vi "Class Loading Progress.vi"(8 "error in (no error)":errorcluster, 10 "Progress (%)":T1 scale=0.0..100.0, 11 "Test Caller Actor in":refnum<class "Test Caller Actor.lvclass">) -> (0 "error out":errorcluster, 3 "Test Caller Actor out":refnum<class "Test Caller Actor.lvclass">)   [LabVIEW 2023, in "Test Caller Actor.lvlib" / "Test Caller Actor.lvclass"]
uses:
  Test Caller Actor.lvclass
  Test Caller Actor.lvclass/Test Caller Actor.ctl
  Class Loader/Class Loader/Loading Progress.ctl
  Class Loader/Class Loader/Class Loader.lvclass
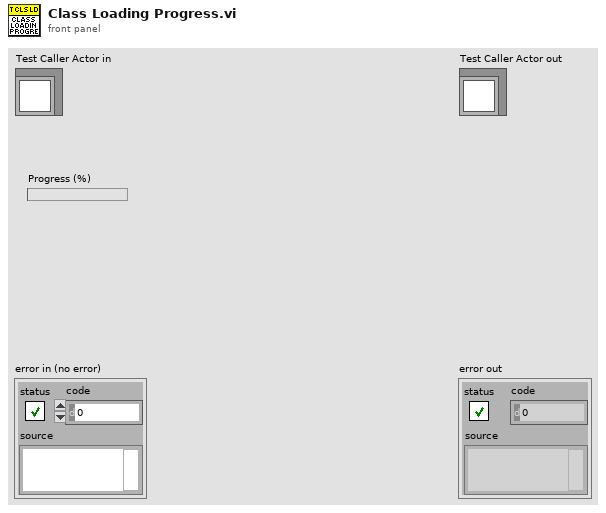
[diagram p1: front panel]
types:
  T1 = typedef "Class Loader.lvlib/Class Loader.lvclass/Loading Progress.ctl" = dbl
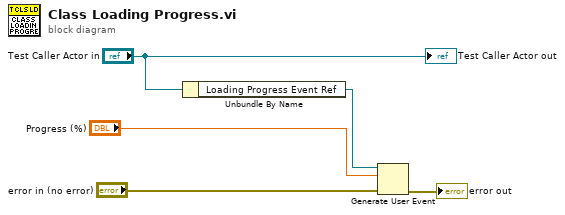
[diagram p0: block diagram]
diagram:
  n1 = Unbundle By Name("Test Caller Actor in") -> ("Loading Progress Event Ref"=w3:refnum<user-event>)
  n2 = Generate User Event(user event=w3, event data cluster="Progress (%)", error in="error in (no error)") -> (error out=→"error out":errorcluster)  [unwired: 1 in, 1 out]
  "Test Caller Actor out" <- "Test Caller Actor in"
